vi "DSF.Engine.Plugin.Initialize.vi"(8 "error in (no error)":errorcluster, 11 "GE Reflective Memory Plugin in":refnum<class "DSF.Plugin.GE Reflective Memory.lvclass">) -> (0 "error out":errorcluster, 3 "GE Reflective Memory Plugin out":refnum<class "DSF.Plugin.GE Reflective Memory.lvclass">)   [LabVIEW 2017, in "DSF.Plugin.GE Reflective Memory.lvclass"]
uses:
  DSF.Plugin.GE Reflective Memory.lvclass
  Engine/Classes/Plugin/DSF.Engine.Plugin.lvclass
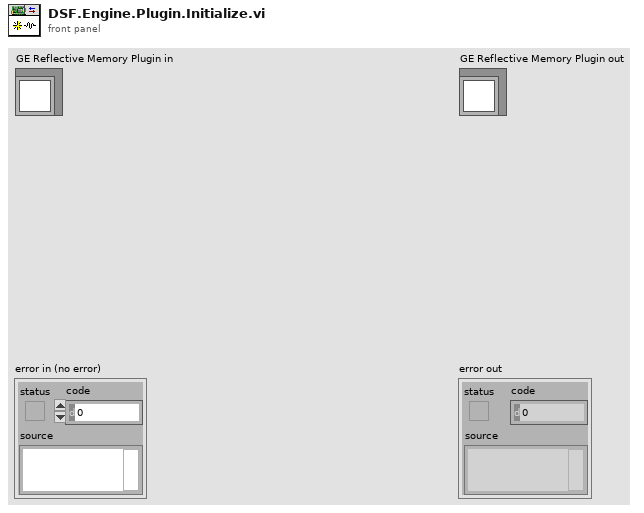
[diagram p1: front panel]
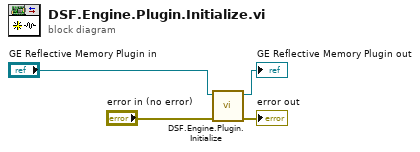
[diagram p0: block diagram]
diagram:
  n1 = call-parent "DSF.Engine.Plugin.Initialize.vi"("error in (no error)"="error in (no error)", "Plugin in"="GE Reflective Memory Plugin in") -> ("error out"=→"error out":errorcluster, "Plugin out"=→"GE Reflective Memory Plugin out":refnum<class "DSF.Plugin.GE Reflective Memory.lvclass">)  [unwired: 8 in]
